vi "AlliGator Load Single Gate Image from SS2 Dataset.vi"(6 "Action":T1, 8 "error in (no error)":errorcluster, 10 "File Info":variant, 11 "Gate Index":i32) -> (0 "error out":errorcluster, 1 "Data 2":sgl[][](array[numeric]), 3 "Data 1":sgl[][](array[numeric]))   [LabVIEW 2021, in "AlliGator Files.lvlib"]
doc: "Loads single gate image from SS2 HDF5 dataset."
uses:
  AlliGator Files.lvlib
  HDF5/AlliGator FLI Image Stack Action.ctl
  SwissSPAD/SS2 Extended Dataset Information.ctl
  SwissSPAD/SS2 File Information.ctl
  SwissSPAD/SS2 FPGA Parameters.ctl
  SwissSPAD/SS2 DAQ Parameters.ctl
  SwissSPAD/SS2 Data Information.ctl
  SwissSPAD/SwissSPAD 8-bit Frames Read.ctl
  7781b2cd-2dca-4692-b5a4-bb2682961437.vi
  Utilities/Logical Processors Used.vi
  SwissSPAD/SwissSPAD.lvlib
  <vilib>/addons/h5labview2/group/H5G.lvlib
  <vilib>/addons/h5labview2/file/H5F.lvlib
  HDF5/AlliGator HDF5.lvlib
panel:
  # "see the AlliGator License on the block diagram (Ctrl+E or Window:Show Block Diagram)"
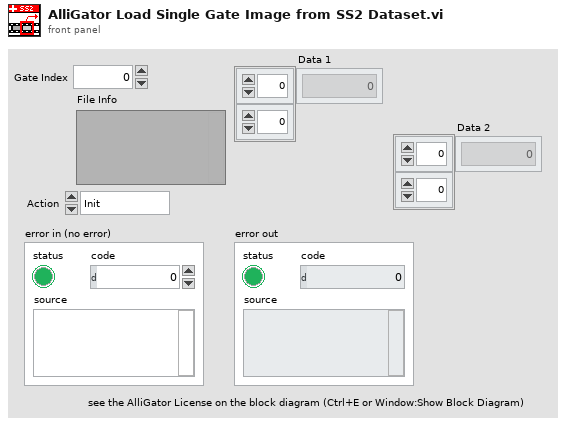
[diagram p1: front panel]
types:
  T1 = typedef "AlliGator HDF5.lvlib/AlliGator FLI Image Stack Action.ctl" = enum16{"Init", "Get Image", "Close"}
  T2 = typedef "SwissSPAD.lvlib/SS2 Extended Dataset Information.ctl" = cluster{"File Path":path, "Swiss SPAD File Information":T3}
  T3 = typedef "SwissSPAD.lvlib/SS2 File Information.ctl" = cluster{"File Version":string, "FPGA Parameters":T4, "DAQ Parameters":T5, "Data Information":T6, "SS2 Frame Selection":T7}
  T4 = typedef "SwissSPAD.lvlib/SS2 FPGA Parameters.ctl" = cluster{"gs_no_shift":i32, "gs_no_shift_adj_1":u32, "gs_no_shift_adj_2":u32, "gs_no_shift_adj_3":u32, "gs_psincdec_0":i32, "gs_psincdec_1":u32, "gs_psincdec 2":u32, "gs_psincdec 3":u32}
  T5 = typedef "SwissSPAD.lvlib/SS2 DAQ Parameters.ctl" = cluster{"Pixel X":i32, "Pixel Y":i32, "# Gate Set":i32, "Bitness":i32, "Gate Offset":i32, "# Gate Positions":i32, "# Exposures/Frame ":i32, "Gate Step":dbl[unit], "Shutter Mode":string, "Laser Frequency":dbl[unit], "Gate Width":dbl[unit]}
  T6 = typedef "SwissSPAD.lvlib/SS2 Data Information.ctl" = cluster{"Sample Description":string, "Author":string, "Software Name":string, "Software Version":string, "Firmware Name":string, "Firmware Version":string}
  T7 = typedef "SwissSPAD.lvlib/SwissSPAD 8-bit Frames Read.ctl" = cluster{"Frame 1":bool, "Frame 2":bool, "Frame 3":bool, "Frame 4":bool}
  T8 = typedef "hid_t.ctl" = i64
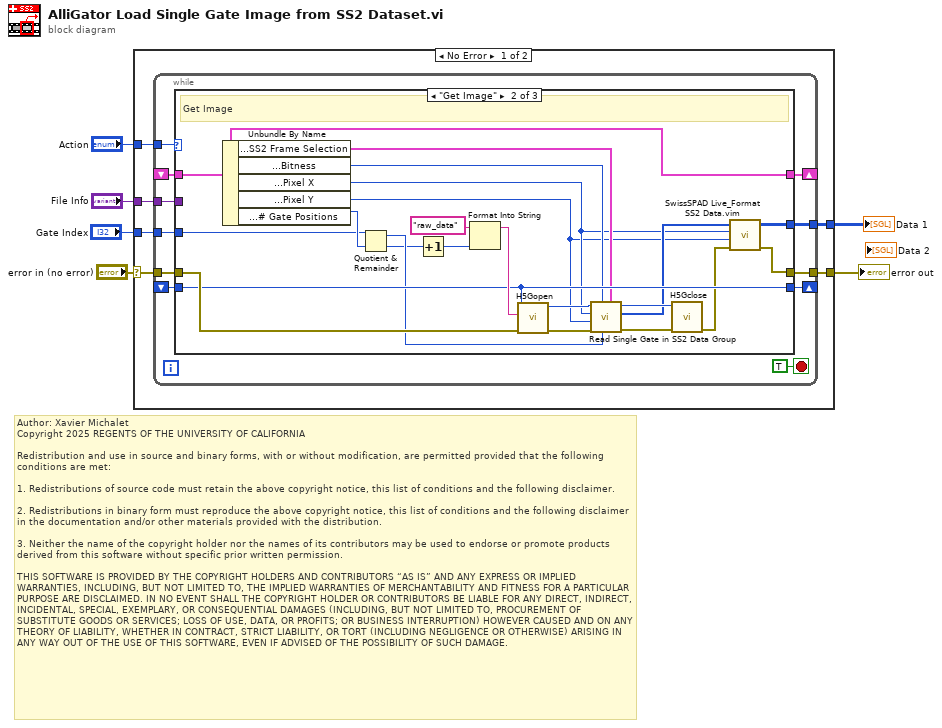
[diagram p0: block diagram]
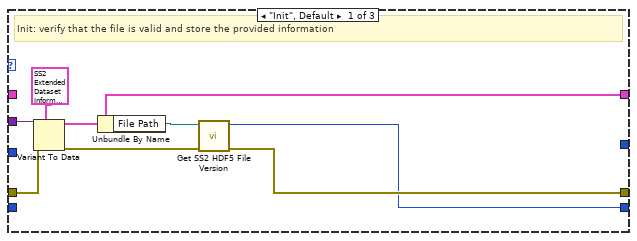
[diagram p2: hidden frame]
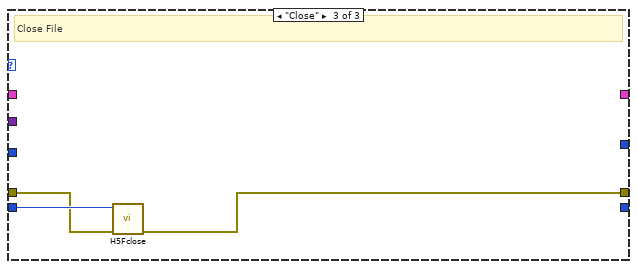
[diagram p3: hidden frame]
diagram:
  # "Author: Xavier Michalet\nCopyright 2025 REGENTS OF THE UNIVERSITY OF CALIFORNIA\n\nRedistribution and use in source and binary forms, with or without modification, are permitted provided that the following conditions are met:\n\n1. Redistributions of source code must retain the above copyright notice, this list of conditions and the following disclaimer.\n\n2. Redistributions in binary form must reproduce the above copyright notice, this list of conditions and the following disclaimer in the documentation and/or other materials provided with the distribution.\n\n3. Neither the name of the copyright holder nor the names of its contributors may be used to endorse or promote products derived from this software without specific prior written permission.\n\nTHIS SOFTWARE IS PROVIDED BY THE COPYRIGHT HOLDERS AND CONTRIBUTORS “AS IS” AND ANY EXPRESS OR IMPLIED WARRANTIES, INCLUDING, BUT NOT LIMITED TO, THE IMPLIED WARRANTIES OF MERCHANTABILITY AND FITNESS FOR A PARTICULAR PURPOSE ARE DISCLAIMED. IN NO EVENT SHALL THE COPYRIGHT HOLDER OR CONTRIBUTORS BE LIABLE FOR ANY DIRECT, INDIRECT, INCIDENTAL, SPECIAL, EXEMPLARY, OR CONSEQUENTIAL DAMAGES (INCLUDING, BUT NOT LIMITED TO, PROCUREMENT OF SUBSTITUTE GOODS OR SERVICES; LOSS OF USE, DATA, OR PROFITS; OR BUSINESS INTERRUPTION) HOWEVER CAUSED AND ON ANY THEORY OF LIABILITY, WHETHER IN CONTRACT, STRICT LIABILITY, OR TORT (INCLUDING NEGLIGENCE OR OTHERWISE) ARISING IN ANY WAY OUT OF THE USE OF THIS SOFTWARE, EVEN IF ADVISED OF THE POSSIBILITY OF SUCH DAMAGE."
  n1 = case shown="No Error" "error in (no error)" {
    selector: "error in (no error)" -> [w11 w57]
    tunnel: [w10 w57] -> w5
    tunnel: "Action" -> [w12 _]
    tunnel: "File Info" -> [w9 _]
    tunnel: "Gate Index" -> [w8 _]
    tunnel: [w7 _] -> w1
    frame No Error {
      n2 = while {
        tunnel: w12 -> [w22]
        tunnel: w11 -> [w21]
        tunnel: [w20] -> w10
        tunnel: w9 -> [w19]
        tunnel: w8 -> [w18]
        shift-right: [w16] -> _
        shift-left: _ -> [w17]
        tunnel: [w15] -> w7
        shift-right: [w14] -> _
        shift-left: _ -> [w13]
        stop <- TRUE stop-if-true
        n3 = case shown="\"Get Image\"" w22 {
          tunnel: w21 -> [w30 w49 w54]
          tunnel: [w26 w43 w55] -> w20
          tunnel: w19 -> [w31 _ _]
          tunnel: w18 -> [_ w37 _]
          tunnel: w17 -> [_ w46 w56]
          tunnel: [w25 w46 _] -> w16
          tunnel: [_ w42 _] -> w15
          tunnel: [w24 w34 _] -> w14
          tunnel: w13 -> [_ w34 _]
          frame "Init", Default {
            # "Init: verify that the file is valid and store the provided information"
            n4 = Variant To Data(error in=w30, type=T2 {"File Path"=path "", "Swiss SPAD File Information"={"File Version"="", "FPGA Parameters"={"gs_no_shift"=0, "gs_no_shift_adj_1"=0, "gs_no_shift_adj_2"=0, "gs_no_shift_adj_3"=0, "gs_psincdec_0"=0, "gs_psincdec_1"=0, "gs_psincdec 2"=0, "gs_psincdec 3"=0}, "DAQ Parameters"={"Pixel X"=0, "Pixel Y"=0, "# Gate Set"=0, "Bitness"=0, "Gate Offset"=0, "# Gate Positions"=0, "# Exposures/Frame "=0, "Gate Step"=0.0, "Shutter Mode"="", "Laser Frequency"=0.0, "Gate Width"=0.0}, "Data Information"={"Sample Description"="", "Author"="", "Software Name"="", "Software Version"="", "Firmware Name"="", "Firmware Version"=""}, "SS2 Frame Selection"={"Frame 1"=FALSE, "Frame 2"=FALSE, "Frame 3"=FALSE, "Frame 4"=FALSE}}} ("Extended SS2 FLI Dataset Information"), Variant=w31) -> (data=w24:T2, error out=w27:errorcluster)
            n5 = Unbundle By Name(w24) -> ("File Path"=w28:path)
            n6 = call "Get SS2 HDF5 File Version.vi"("error in (no error)"=w27, "path in"=w28) -> ("error out"=w26:errorcluster, "ref out"=w25:i32)  [unwired: 7 in, 1 out]
          }
          frame "Get Image" {
            # "Get Image"
            n7 = Unbundle By Name(w34) -> ("Swiss SPAD File Information.SS2 Frame Selection"=w40:T7, "Swiss SPAD File Information.DAQ Parameters.Bitness"=w41:i32, "Swiss SPAD File Information.DAQ Parameters.Pixel X"=w33:i32, "Swiss SPAD File Information.DAQ Parameters.Pixel Y"=w32:i32, "Swiss SPAD File Information.DAQ Parameters.# Gate Positions"=w39:i32)
            n8 = Quotient & Remainder(x=w37, y=w39) -> (x-y*floor(x/y)=w38:i32, floor(x/y)=w36:i32)
            n9 = Increment(x=w36) -> (x+1=w35:i32)
            n10 = Format Into String(initial string="raw_data", w35) -> (resulting string=w53:string)  [unwired: 2 in, 1 out]
            n11 = call <vilib>:"H5Gopen.vi"("error in (no error)"=w49, "name"=w53, "ref in"=w46) -> ("error out"=w51:errorcluster, "group out"=w48:T8)  [unwired: 7 in]
            n12 = call "Read Single Gate in SS2 Data Group.vi"("SS2 8-bit Frame Selection"=w40, "Gate Idx"=w38, "Bitness"=w41, "error in (no error)"=w51, "Pixel Y"=w32, "Pixel X"=w33, "group in"=w48) -> ("error out"=w50:errorcluster, "Data"=w45:u16[], "group out"=w47:T8)  [unwired: 2 out]
            n13 = call <vilib>:"H5Gclose.vi"("error in (no error)"=w50, "group in"=w47) -> ("error out"=w44:errorcluster)  [unwired: 9 in]
            n14 = call "SwissSPAD Live_Format SS2 Data.vim"("Error In"=w44, "Y Resolution"=w32, "X Resolution"=w33, "Flattened Image"=w45) -> ("Error Out"=w43:errorcluster, "Image out"=w42:u16[][])  [unwired: 6 in]
          }
          frame "Close" {
            # "Close File"
            n15 = call <vilib>:"H5Fclose.vi"("error in (no error)"=w54, "ref"=w56) -> ("error out"=w55:errorcluster)  [unwired: 9 in]
          }
        }
      }
    }
    frame Error {
    }
  }
  "Data 1" <- w1
  "error out" <- w5
